vi "Averaged_Rot_Measure_Main_v2.vi"() -> ()   [LabVIEW 2021]
uses:
  Config_File_Paths.ctl
  ZI_Data.ctl
  <vilib>/Analysis/baseanly.llb/Mean (DBL).vi
  <vilib>/Utility/file.llb/Write Delimited Spreadsheet (DBL).vi
  <vilib>/measure/maspectr.llb/FFT Spectrum (Real-Im) for 1 Chan.vi
  <vilib>/Analysis/NI_AALPro.lvlib
  <vilib>/measure/NI_MAPro.lvlib
  <vilib>/Analysis/NI_AALBase.lvlib
panel:
  out "averaged rotation":cluster{"Time":dbl[], "X":dbl[]}[](graph)
  out "single differ 2":cluster{"Time":dbl[], "X":dbl[]}[](graph)
  out "Possible Mismatch In Phase (?)":bool
  out "Enough Points (?)":bool
  out "Trig Out Found(?)":bool
  out "Meter":dbl(knob) scale=-15.0..15.0
  out "single abs\nspectrum":waveform(dbl)(graph)
  out "averaged spectrum":waveform(dbl)[](graph)
  out "single rot \nspectrum":waveform(dbl)[](graph)
  out "single differ":cluster{"Time":dbl[], "X":dbl[]}[](graph)
  out "single abs":cluster{"Time":dbl[], dbl[]}(graph)
  out "single rot":cluster{"Time":dbl[], "X":dbl[]}[](graph)
  in  "Resource Address":T1={"ZI Address"="DEV714", "VISA Keithley"="KEITHLEY", "VISA Arduino PG"="Arduino_PGen"}
  in  "error in":errorcluster
  in  "Config files paths":T2={"ZI config file (.ini)"="Config_Ver_1\\Zurich_params.ini", "Keithley config file (.ini)"="Config_Ver_1\\Keithley_params.ini", "Arduino config file (.ini)"="Config_Ver_1\\pulse_sequence.ini"}
  in  "Time unit":string(combo)="ms"
  out "loading":dbl(slide) scale=0.0..100.0
  in  "Number of averages":i32=1
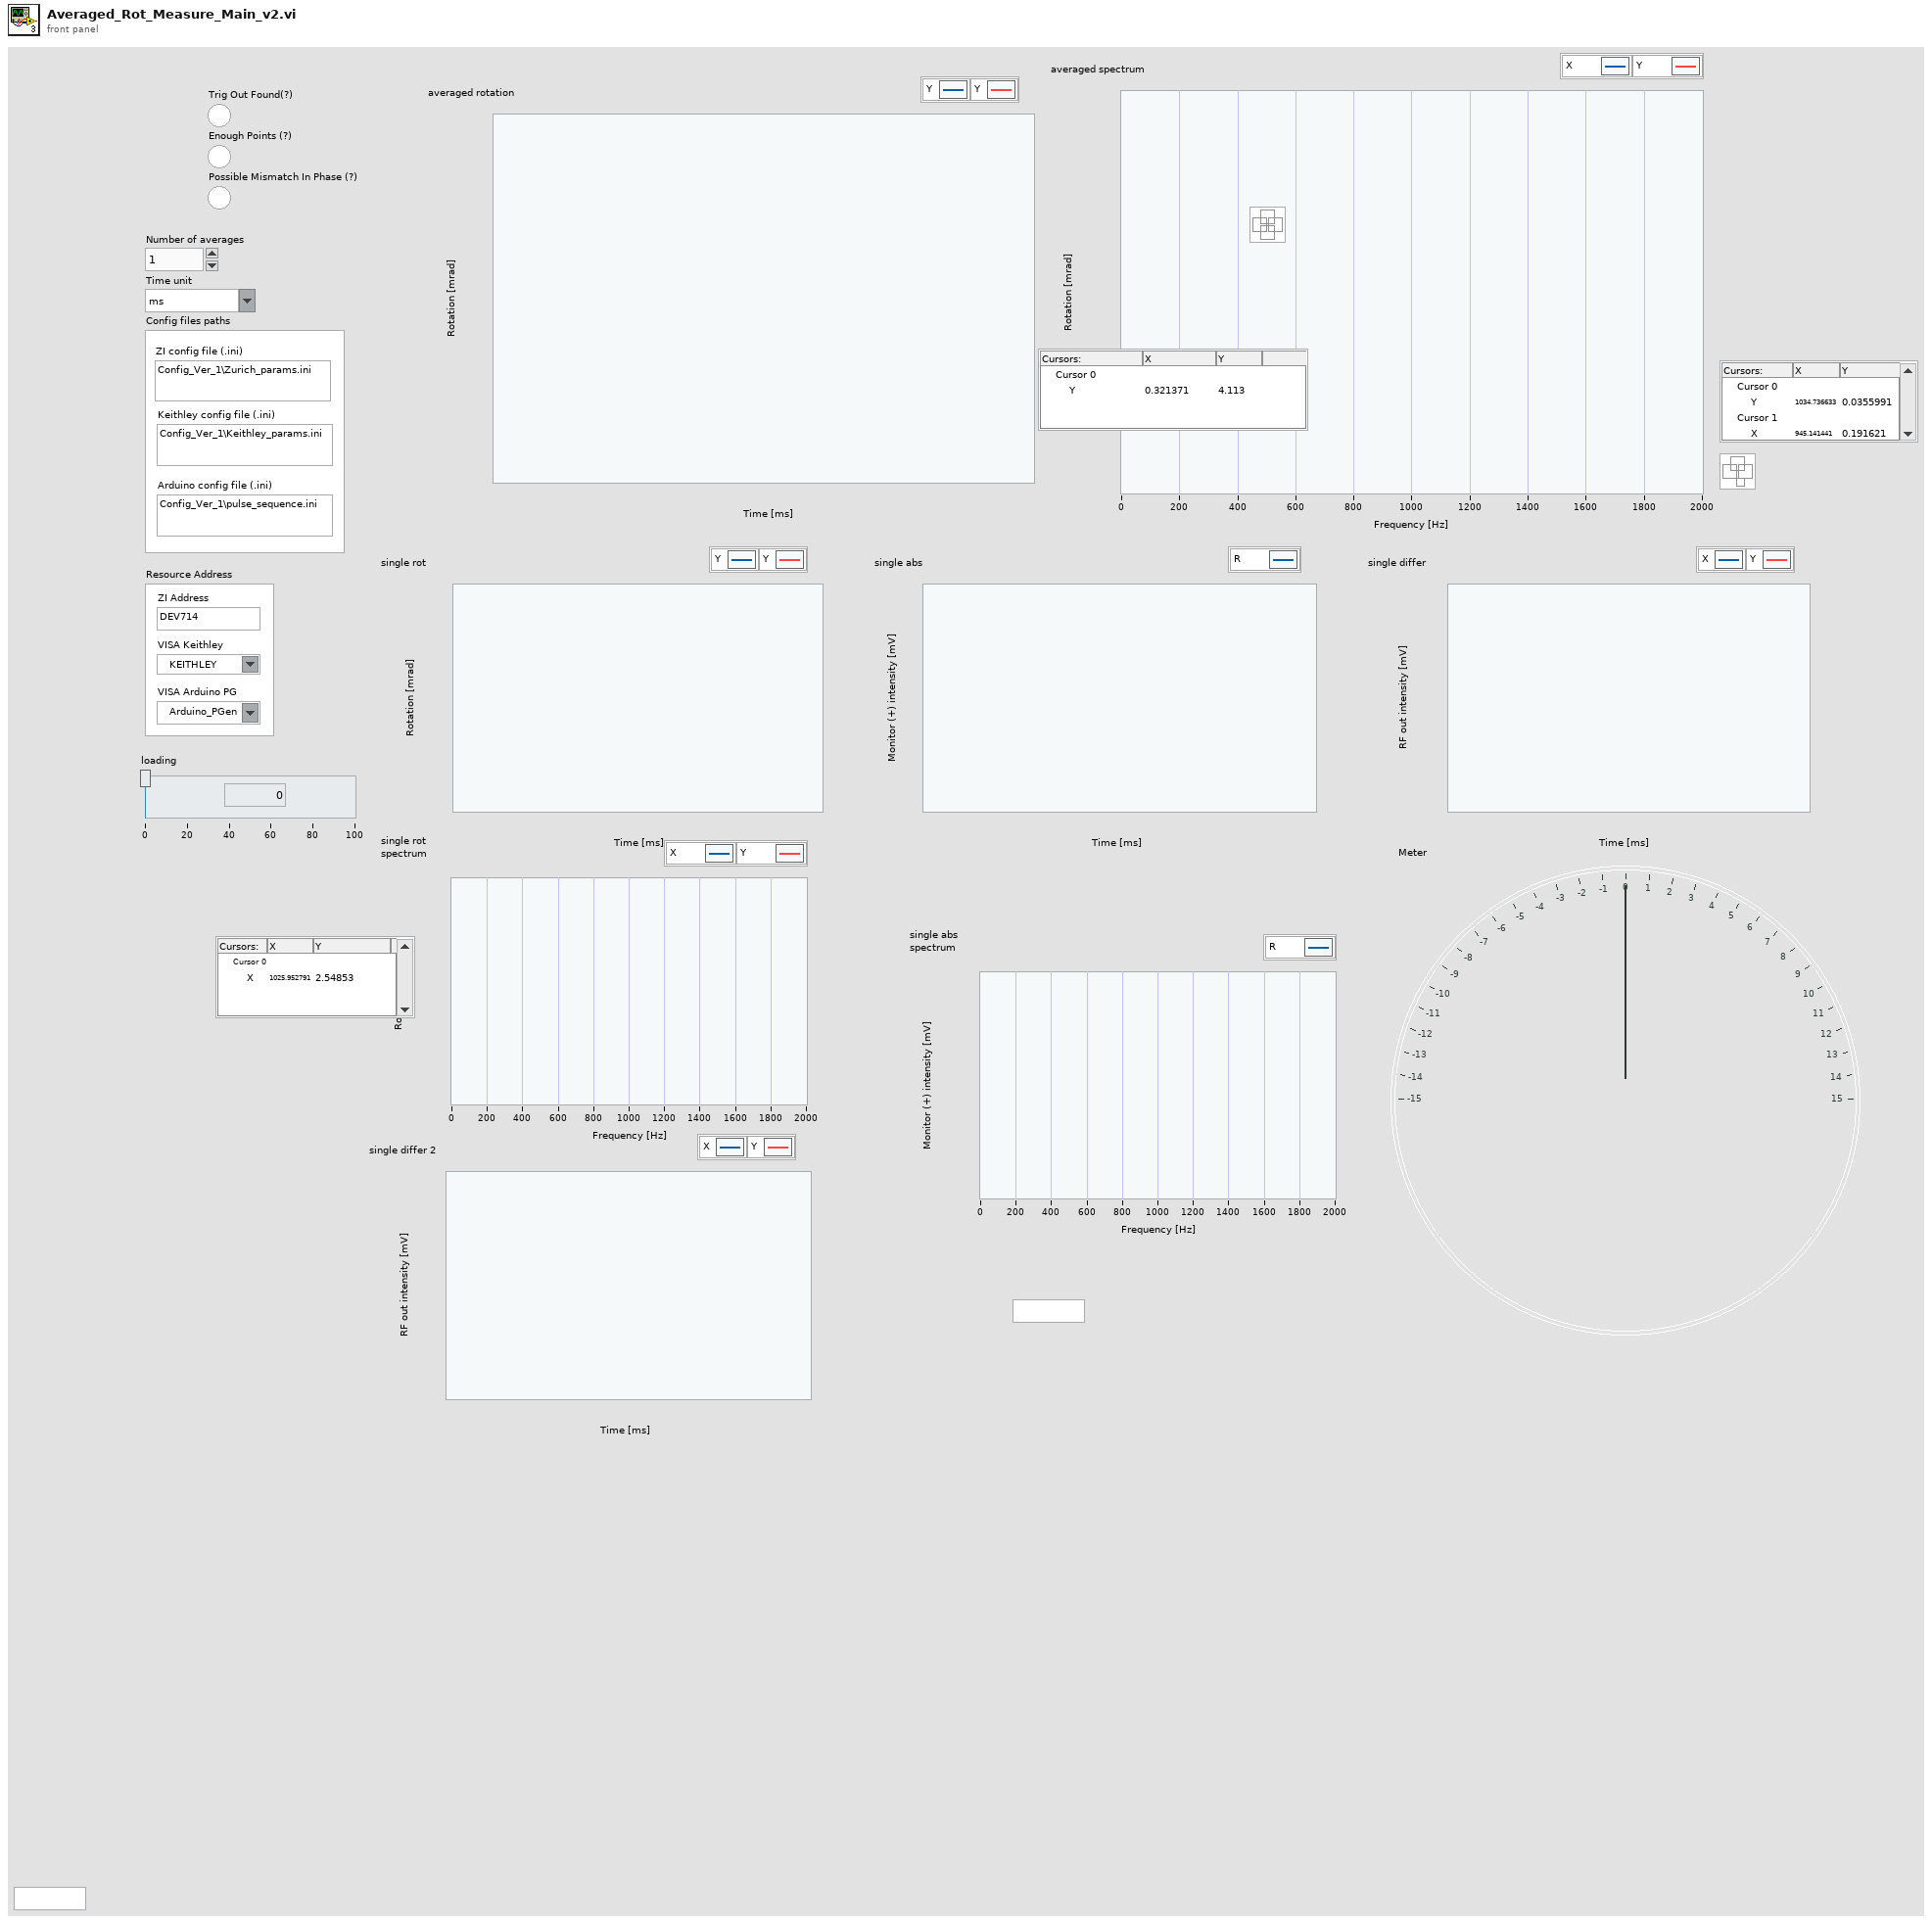
[diagram p1: front panel]
types:
  T1 = cluster{"ZI Address":string, "VISA Keithley":refnum<visa-resource-name>, "VISA Arduino PG":refnum<visa-resource-name>}
  T2 = typedef "Config_File_Paths.ctl" = cluster{"ZI config file (.ini)":string, "Keithley config file (.ini)":string, "Arduino config file (.ini)":string}
  T3 = typedef "ZI_Data.ctl" = cluster{"R":dbl[], "Theta":dbl[], "X":dbl[], "Y":dbl[], "AuxIn0":dbl[], "AuxIn1":dbl[], "Frequency":dbl[], "DIO":dbl[], "Time":dbl[]}
  T4 = typedef "Resources.ctl" = cluster{"ZI Handle":T5, "ZI ModHandle":T6, "VISA arduino":refnum<visa-resource-name>, "VISA Keithley":refnum<visa-resource-name>}
  T5 = typedef "Zurich Instruments LabOne.lvlib/ziTypeHandle.ctl" = cluster{"handleValid":bool, "Conn":u64, "Path Prefix":string, "Handle":u64, "Connected":bool, "Clockbase(s)":dbl}
  T6 = typedef "Zurich Instruments LabOne.lvlib/ziTypeModHandle.ctl" = cluster{"handleValid":bool, "Conn":u64, "ModHandle":u64, "moduleID":string, "Path Prefix":string}
  T7 = typedef "Cutted_Data.ctl" = cluster{"X":dbl[], "Y":dbl[], "Time":dbl[]}
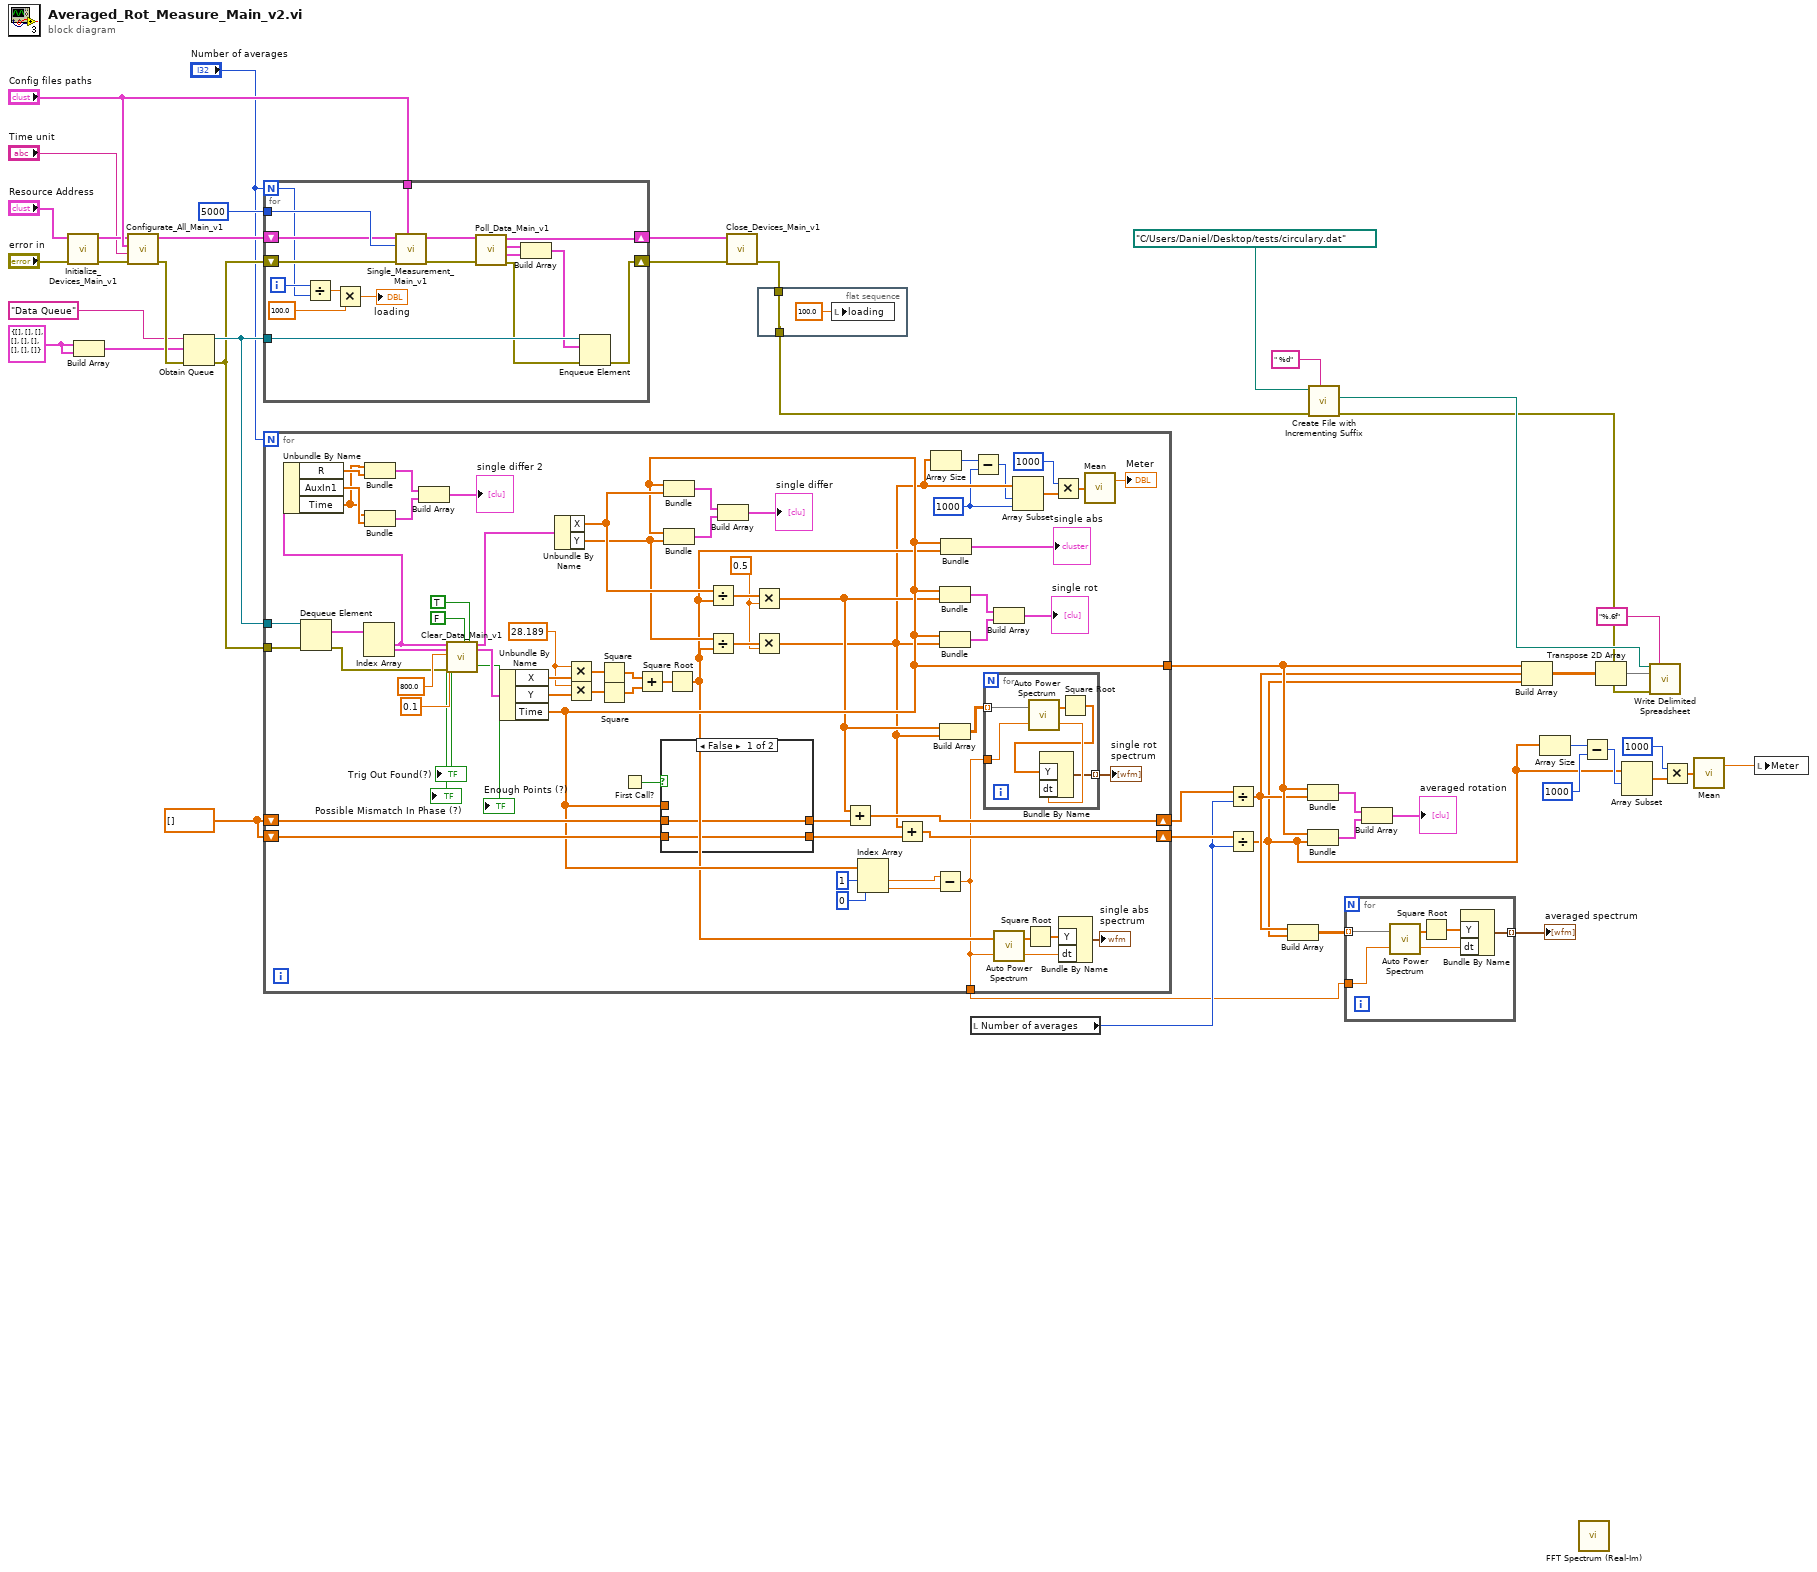
[diagram p0: block diagram]
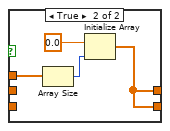
[diagram p2: hidden frame]
diagram:
  w30 = dbl[] []
  w34 = T3 {"R"=[], "Theta"=[], "X"=[], "Y"=[], "AuxIn0"=[], "AuxIn1"=[], "Frequency"=[], "DIO"=[], "Time"=[]} ("ZI Data")
  n1 = call "Initialize_Devices_Main_v1.vi"("error in"="error in", "Resource Address"="Resource Address") -> ("error out"=w38:errorcluster, "Resources"=w39:T4)  [unwired: 8 in]
  n2 = Build Array(w34, w34) -> (w33:T3[])
  n3 = call "Configurate_All_Main_v1.vi"("error in"=w38, "Time unit"="Time unit", "Config files paths"="Config files paths", "Resources in"=w39) -> ("error out"=w36:errorcluster, "Resources out"=w44:T4)  [unwired: 4 in, 2 out]
  n4 = Obtain Queue(name (unnamed)="Data Queue", element data type=w33, error in (no error)=w36) -> (queue out=w32:refnum<queue>, error out=w31:errorcluster)  [unwired: 2 in, 1 out]
  n5 = for {
    N: "Number of averages" -> [w56]
    shift-right: [w58] -> w45
    shift-left: w44 -> [w62]
    shift-right: [w47] -> w46
    shift-left: w31 -> [w61]
    tunnel: "Config files paths" -> [w64]
    tunnel: u64 5000 ("Timeout [ms]") -> [w63]
    tunnel: w32 -> [w52]
    i -> [w57]
    n6 = Divide(x=w57, y=w56) -> (x/y=w55:dbl)
    n7 = Multiply(x=w55, y=100.0) -> (x*y=→"loading":dbl)
    n8 = call "Single_Measurement_Main_v1.vi"("Config files paths"=w64, "error in"=w61, "Timeout [ms]"=w63, "Resources In"=w62) -> ("error out"=w59:errorcluster, "Resources Out"=w60:T4)  [unwired: 6 in]
    n9 = call "Poll_Data_Main_v1.vi"("error in"=w59, "Resources in"=w60) -> ("error out"=w48:errorcluster, "ZI Data 3"=w50:T3, "ZI Data 0"=w51:T3, "Resources out"=w58:T4)  [unwired: 6 in]
    n10 = Build Array(w51, w50) -> (w49:T3[])
    n11 = Enqueue Element(queue=w52, element=w49, error in (no error)=w48) -> (error out=w47:errorcluster)  [unwired: 1 in, 2 out]
  }
  n12 = for {
    N: "Number of averages" -> [_]
    tunnel: w32 -> [w134]
    tunnel: w31 -> [w133]
    shift-right: [w118] -> w27
    shift-left: w30 -> [w122]
    shift-right: [w117] -> w28
    shift-left: w30 -> [w121]
    tunnel: [w103] -> w17
    tunnel: [w86] -> w10
    w81 = 1000 ("length")
    w105 = 0.5
    w65 = 28.189
    n13 = Dequeue Element(queue=w134, error in (no error)=w133) -> (element=w132:T3[], error out=w128:errorcluster)  [unwired: 1 in, 2 out]
    n14 = Index Array(array=w132) -> (element #1=w72:T3, element #2=w131:T3)  [unwired: 2 in]
    n15 = Unbundle By Name(w72) -> ("R"=w68:dbl[], "AuxIn1"=w67:dbl[], "Time"=w66:dbl[])
    n16 = Bundle("Time"=w66, "R"=w68) -> (w71:cluster{"Time":dbl[], "R":dbl[]})  [unwired: 1 in]
    n17 = Bundle("Time"=w66, "AuxIn1"=w67) -> (w70:cluster{"Time":dbl[], "AuxIn1":dbl[]})  [unwired: 1 in]
    n18 = Build Array(w71, w70) -> (→"single differ 2":cluster{"Time":dbl[], "AuxIn1":dbl[]}[])
    n19 = call "Clear_Data_Main_v1.vi"("ZI Data 0"=w72, "ZI Data 3"=w131, "Time Of Collected Data (ms)"=800.0, "Crosstalk Tolerance"=0.1, "error in"=w128, "Fixed Number Of Points"=FALSE, "Check Phase Mismatch"=TRUE) -> ("Trig Out Found(?)"=→"Trig Out Found(?)":bool, "Enough Points (?)"=→"Enough Points (?)":bool, "Possible Mismatch In Phase (?)"=→"Possible Mismatch In Phase (?)":bool, "Cutted Data"=w125:T7, "Cutted Data 3"=w124:T7)  [unwired: 7 in, 1 out]
    n20 = Unbundle By Name(w124) -> ("X"=w108:dbl[], "Y"=w109:dbl[], "Time"=w103:dbl[])
    n21 = Unbundle By Name(w125) -> ("X"=w110:dbl[], "Y"=w97:dbl[])
    n22 = Multiply(x=w65, y=w108) -> (x*y=w93:dbl[])
    n23 = Multiply(x=w65, y=w109) -> (x*y=w92:dbl[])
    n24 = Square(x=w93) -> (x^2=w95:dbl[])
    n25 = Square(x=w92) -> (x^2=w94:dbl[])
    n26 = First Call?() -> (First Call?: T/F=w123:bool)
    n27 = Add(x=w95, y=w94) -> (x+y=w96:dbl[])
    n28 = case shown="False" w123 {
      tunnel: w103 -> [_ w146]
      tunnel: w122 -> [w142 _]
      tunnel: [w142 w143] -> w119
      tunnel: [w141 w143] -> w120
      tunnel: w121 -> [w141 _]
      frame False {
      }
      frame True {
        n29 = Array Size(array=w146) -> (size(s)=w144:i32)
        n30 = Initialize Array(0.0 ("element"), w144) -> (w143:dbl[])
      }
    }
    n31 = Bundle("Time"=w103, "X"=w110) -> (w113:cluster{"Time":dbl[], "X":dbl[]})  [unwired: 1 in]
    n32 = Bundle("Time"=w103, "Y"=w97) -> (w112:cluster{"Time":dbl[], "Y":dbl[]})  [unwired: 1 in]
    n33 = Square Root(x=w96) -> (sqrt(x)=w87:dbl[])
    n34 = Divide(x=w110, y=w87) -> (x/y=w107:dbl[])
    n35 = Divide(x=w97, y=w87) -> (x/y=w106:dbl[])
    n36 = Build Array(w113, w112) -> (→"single differ":cluster{"Time":dbl[], "Y":dbl[]}[])
    n37 = Multiply(x=w107, y=w105) -> (x*y=w90:dbl[])
    n38 = Multiply(x=w106, y=w105) -> (x*y=w82:dbl[])
    n39 = Add(x=w90, y=w119) -> (x+y=w118:dbl[])
    n40 = Index Array(array=w103, index #1=1 ("index"), index #2=0 ("index")) -> (element #1=w100:dbl, element #2=w99:dbl)
    n41 = Add(x=w82, y=w120) -> (x+y=w117:dbl[])
    n42 = Array Size(array=w82) -> (size(s)=w80:i32)
    n43 = Subtract(x=w100, y=w99) -> (x-y=w86:dbl)
    n44 = Bundle("Time"=w103, w90) -> (w116:cluster{"Time":dbl[], dbl[]})  [unwired: 1 in]
    n45 = Bundle("Time"=w103, w82) -> (w115:cluster{"Time":dbl[], dbl[]})  [unwired: 1 in]
    n46 = Build Array(w90, w82) -> (w104:dbl[][])
    n47 = Bundle("Time"=w103, w87) -> (→"single abs":cluster{"Time":dbl[], dbl[]})  [unwired: 1 in]
    n48 = Subtract(x=w80, y=w81) -> (x-y=w79:i32)
    n49 = for {
      tunnel: w104 -> [w140] mode=indexing
      tunnel: w86 -> [w139]
      tunnel: [w137] -> w98 mode=indexing
      n50 = call <vilib>:"Auto Power Spectrum.vi"("dt"=w139, "Signal (V)"=w140) -> ("df"=w138:dbl, "Power Spectrum (V^2 rms)"=w136:dbl[])
      n51 = Square Root(x=w136) -> (sqrt(x)=w135:dbl[])
      n52 = Bundle By Name("Y"=w135, "dt"=w138) -> (w137:waveform(dbl))  [unwired: 1 in]
    }
    "single rot \nspectrum" <- w98
    n53 = Build Array(w116, w115) -> (→"single rot":cluster{"Time":dbl[], dbl[]}[])
    n54 = call <vilib>:"Auto Power Spectrum.vi"("dt"=w86, "Signal (V)"=w87) -> ("df"=w88:dbl, "Power Spectrum (V^2 rms)"=w89:dbl[])
    n55 = Array Subset(array=w82, index=w79, length=w81) -> (w78:dbl[])
    n56 = Square Root(x=w89) -> (sqrt(x)=w85:dbl[])
    n57 = Multiply(x=1000, y=w78) -> (x*y=w76:dbl[])
    n58 = Bundle By Name("Y"=w85, "dt"=w88) -> (→"single abs\nspectrum":waveform(dbl))  [unwired: 1 in]
    n59 = call-poly <vilib>:"Mean.vi"("X"=w76) -> ("mean"=→"Meter":dbl)  [unwired: 1 out]
  }
  n60 = call "Close_Devices_Main_v1.vi"("error in"=w46, "Resources in"=w45) -> ("error out"=w12:errorcluster)  [unwired: 9 in]
  n61 = flat-sequence {
    tunnel: [w147] -> w11
    tunnel: w12 -> [w147]
    frame #0 {
      n62 = local write "loading"(100.0 ("loading")) -> ()
    }
  }
  n63 = local read "Number of averages"() -> (w26:i32)
  n64 = Divide(x=w27, y=w26) -> (x/y=w15:dbl[])
  n65 = Divide(x=w28, y=w26) -> (x/y=w3:dbl[])
  n66 = Build Array(w15, w3) -> (w14:dbl[][])
  n67 = Bundle("Time"=w17, w15) -> (w24:cluster{"Time":dbl[], dbl[]})  [unwired: 1 in]
  n68 = Bundle("Time"=w17, w3) -> (w25:cluster{"Time":dbl[], dbl[]})  [unwired: 1 in]
  n69 = call <vilib>:"Create File with Incrementing Suffix.vi"("format string (\" (%d)\")"=" %d" ("format string (\" (%d)\")"), "error in (no error)"=w11, "file path"=path "C:/Users/Daniel/Desktop/tests/circulary.dat") -> ("error out"=w16:errorcluster, "actual path"=w18:path)  [unwired: 6 in, 1 out]
  n70 = for {
    tunnel: w14 -> [w154] mode=indexing
    tunnel: w10 -> [w153]
    tunnel: [w151] -> w13 mode=indexing
    n71 = call <vilib>:"Auto Power Spectrum.vi"("dt"=w153, "Signal (V)"=w154) -> ("df"=w152:dbl, "Power Spectrum (V^2 rms)"=w150:dbl[])
    n72 = Square Root(x=w150) -> (sqrt(x)=w149:dbl[])
    n73 = Bundle By Name("Y"=w149, "dt"=w152) -> (w151:waveform(dbl))  [unwired: 1 in]
  }
  "averaged spectrum" <- w13
  n74 = Build Array(w24, w25) -> (→"averaged rotation":cluster{"Time":dbl[], dbl[]}[])
  n75 = Build Array(w17, w15, w3) -> (w21:dbl[][])
  n76 = Array Size(array=w3) -> (size(s)=w5:i32)
  n77 = call-poly <vilib>:"FFT Spectrum (Real-Im).vi"() -> ()  [unwired: 7 in, 5 out]
  n78 = Subtract(x=w5, y=1000 ("length")) -> (x-y=w6:i32)
  n79 = Transpose 2D Array(2D array=w21) -> (transposed array=w20:dbl[][])
  n80 = Array Subset(array=w3, index=w6) -> (w7:dbl[])  [unwired: 1 in]
  n81 = call-poly <vilib>:"Write Delimited Spreadsheet.vi"("file path (dialog if empty)"=w18, "format (%.3f)"="%.6f", "2D data"=w20, "error in (no error)"=w16) -> ()  [unwired: 10 in, 2 out]
  n82 = Multiply(x=1000, y=w7) -> (x*y=w9:dbl[])
  n83 = call-poly <vilib>:"Mean.vi"("X"=w9) -> ("mean"=w2:dbl)  [unwired: 1 out]
  n84 = local write "Meter"(w2) -> ()
